vi "Read Measurement.vi"(8 "error in (no error)":errorcluster, 9 "Measurement Type (0: Frequency)":i32(ring) items=["Frequency", "Mean", "Period", "Pulse Duty", "Peak to Peak", "Cycle RMS", "Minimum", "Maximum", "Rise Time", "Fall Time", "Positive Width", "Negative Width", "Amplitude", "Cycle Mean", "High", "Low", "Negative Duty", "Positive Overshoot", "Negative Overshoot", "Cursor Mean", "Burst Width", "Positive Pulse Count", "Negative Pulse Count", "Rising Edge Count", "Falling Edge Count", "Area", "Cycle Area", "RMS", "Cursor RMS"], 10 "Channel (1: Channel 1)":i32(ring)=1 items=["Channel 1"=1, "Channel 2"=2, "Channel 3"=3, "Channel 4"=4], 11 "VISA resource name":refnum<visa-resource-name>) -> (0 "error out":errorcluster, 1 "Units":string, 2 "Measurement":dbl, 3 "VISA resource name out":refnum<visa-resource-name>)   [LabVIEW 2017, in "Tektronix TDS 200 1000 2000 Series.lvlib"]
doc: "Reads a user-specified instrument from the waveform on the selected channel."
uses:
  Tektronix TDS 200 1000 2000 Series.lvlib
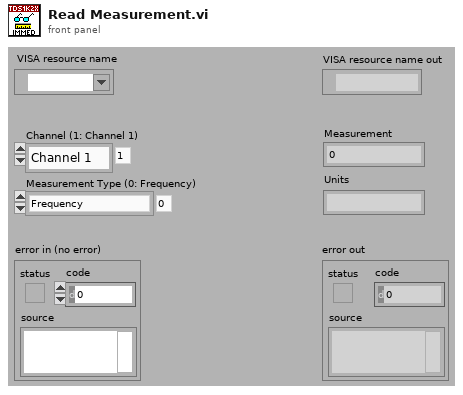
[diagram p1: front panel]
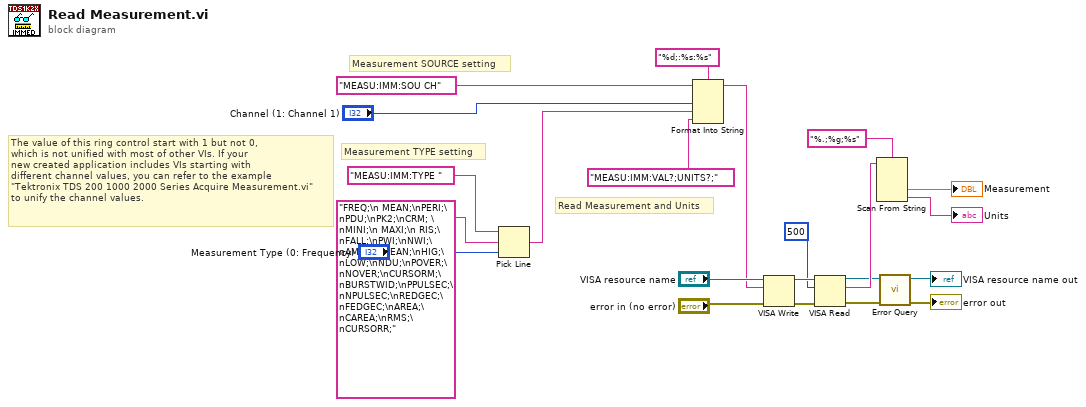
[diagram p0: block diagram]
diagram:
  # "The value of this ring control start with 1 but not 0, \nwhich is not unified with most of other VIs. If your \nnew created application includes VIs starting with \ndifferent channel values, you can refer to the example\n\"Tektronix TDS 200 1000 2000 Series Acquire Measurement.vi\"\nto unify the channel values."
  # "Read Measurement and Units"
  # "Measurement SOURCE setting"
  # "Measurement TYPE setting"
  n1 = Pick Line(string ("")="MEASU:IMM:TYPE ", multi-line string="FREQ;\n MEAN;\nPERI;\nPDU;\nPK2;\nCRM; \nMINI;\n MAXI;\n RIS;\nFALL;\nPWI;\nNWI;\nAMP;\nCMEAN;\nHIG;\nLOW;\nNDU;\nPOVER;\nNOVER;\nCURSORM;\nBURSTWID;\nPPULSEC;\nNPULSEC;\nREDGEC;\nFEDGEC;\nAREA;\nCAREA;\nRMS;\nCURSORR;", line index="Measurement Type (0: Frequency)") -> (output string=w8:string)
  n2 = Format Into String(format string="%d;:%s:%s", initial string="MEASU:IMM:SOU CH" ("string (\"\")"), "Channel (1: Channel 1)", w8, "MEASU:IMM:VAL?;UNITS?;" ("write buffer")) -> (resulting string=w6:string)  [unwired: 1 in, 1 out]
  n3 = VISA Write(VISA resource name="VISA resource name", write buffer=w6, error in (no error)="error in (no error)") -> (VISA resource name out=w20:refnum<visa-resource-name>, error out=w19:errorcluster)  [unwired: 1 out]
  n4 = VISA Read(VISA resource name=w20, byte count=u32 500, error in (no error)=w19) -> (VISA resource name out=w2:refnum<visa-resource-name>, read buffer=w14:string, error out=w3:errorcluster)  [unwired: 1 out]
  n5 = Scan From String(format string="%.;%g;%s", input string=w14) -> (output 1=→"Measurement":dbl, output 2=→"Units":string)  [unwired: 2 in, 5 out]
  n6 = call "Error Query.vi"("error in (no error)"=w3, "VISA resource name"=w2) -> ("error out"=→"error out":errorcluster, "VISA resource name out"=→"VISA resource name out":refnum<visa-resource-name>)  [unwired: 8 out]
